vi "Resize Panel to Pane.vi"(8 "error in (no error)":errorcluster, 10 "NewBnds":T1, 11 "ActorAutoRegPanel In":refnum<class "ActorAutoRegPanel.lvclass">) -> (0 "error out":errorcluster, 3 "ActorAutoRegPanel Out":refnum<class "ActorAutoRegPanel.lvclass">)   [LabVIEW 2015, in "TestActors.lvlib" / "ActorAutoRegPanel.lvclass"]
uses:
  ActorAutoRegPanel.lvclass
  <vilib>/Utility/miscctls.llb/LVRectTypeDef.ctl
  Dialog Box Implementations/OneButtonDialogBox/OneButtonDialogBox.lvclass
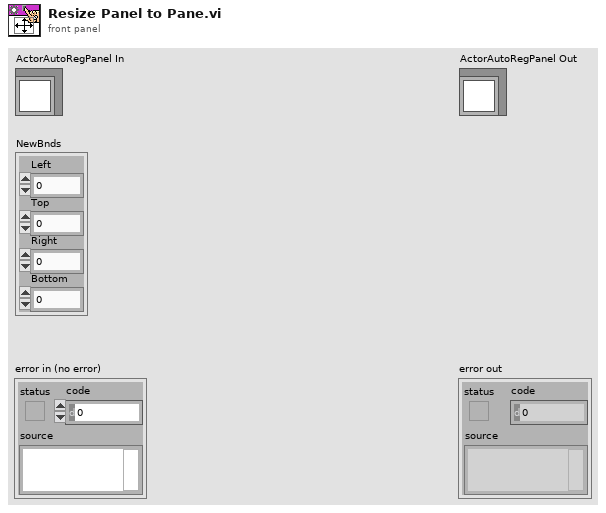
[diagram p1: front panel]
types:
  T1 = typedef "LVRectTypeDef.ctl" = cluster{"Left":i16, "Top":i16, "Right":i16, "Bottom":i16}
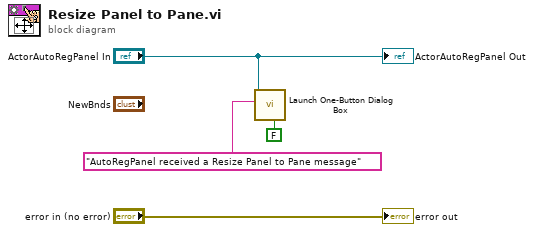
[diagram p0: block diagram]
diagram:
  n1 = call "Launch One-Button Dialog Box.vi"("Modal? (T)"=FALSE, "Message Text"="AutoRegPanel received a Resize Panel to Pane message", "Dialog Launcher"="ActorAutoRegPanel In") -> ()  [unwired: 8 in, 1 out]
  "error out" <- "error in (no error)"
  "ActorAutoRegPanel Out" <- "ActorAutoRegPanel In"
